vi "RaiseForTime-C.vi"(11 "Params":string[][](array[string])) -> ()   [LabVIEW 2018]
uses:
  Framework/Robot Global Data.vi
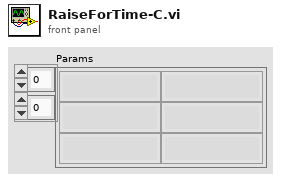
[diagram p1: front panel]
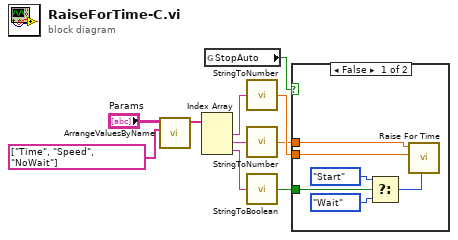
[diagram p0: block diagram]
diagram:
  n1 = call "ArrangeValuesByName.vi"("Names"=string[] ["Time", "Speed", "NoWait"], "Names/Values in"="Params") -> ("Values Out"=w4:string[])  [unwired: 9 in]
  n2 = Index Array(array=w4) -> (element #1=w3:string, element #2=w2:string, element #3=w1:string)  [unwired: 3 in]
  n3 = global read "Robot Global Data.vi" "StopAuto"() -> (w10:bool)
  n4 = call "StringToNumber.vi"("String"=w3) -> ("Output"=w9:dbl)
  n5 = call "StringToNumber.vi"("String"=w2) -> ("Output"=w8:dbl)
  n6 = call "StringToBoolean.vi"("String"=w1) -> ("Output"=w7:bool)
  n7 = case shown="False" w10 {
    tunnel: w9 -> [w11 _]
    tunnel: w8 -> [w12 _]
    tunnel: w7 -> [w14 _]
    frame False {
      n8 = Select(t=enum16{"Start", "Wait"}."Start" ("Synchronization"), s=w14, f=enum16{"Start", "Wait"}."Wait" ("Synchronization")) -> (s? t:f=w13:enum16{"Start", "Wait"})
      n9 = call "Raise For Time.vi"("Synchronization"=w13, "Time"=w11, "Speed"=w12) -> ()  [unwired: 8 in, 1 out]
    }
    frame True {
    }
  }
